vi "3HeClose.vi"(8 "error in (no error)":errorcluster, 11 "VISA resource name":refnum<visa-resource-name>) -> (0 "error out":errorcluster)   [LabVIEW 2018]
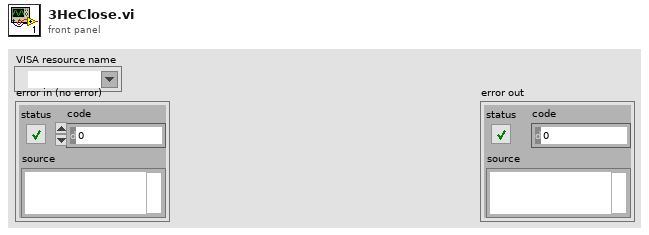
[diagram p1: front panel]
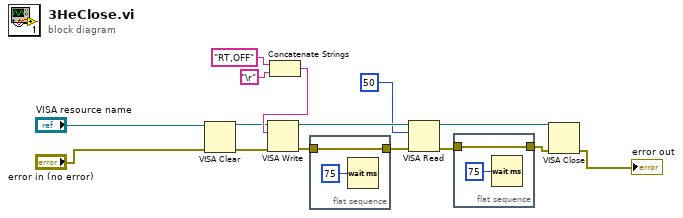
[diagram p0: block diagram]
diagram:
  n1 = VISA Clear(VISA resource name="VISA resource name", error in (no error)="error in (no error)") -> (VISA resource name out=w8:refnum<visa-resource-name>, error out=w9:errorcluster)
  n2 = Concatenate Strings("RT,OFF" ("write buffer"), "\r") -> (w10:string)
  n3 = VISA Write(VISA resource name=w8, write buffer=w10, error in (no error)=w9) -> (VISA resource name out=w14:refnum<visa-resource-name>, error out=w15:errorcluster)  [unwired: 1 out]
  n4 = flat-sequence {
    tunnel: w15 -> [w16]
    tunnel: [w16] -> w13
    frame #0 {
      n5 = Wait (ms)(milliseconds to wait=u32 75) -> ()  [unwired: 1 out]
    }
  }
  n6 = VISA Read(VISA resource name=w14, byte count=u32 50, error in (no error)=w13) -> (VISA resource name out=w3:refnum<visa-resource-name>, error out=w5:errorcluster)  [unwired: 2 out]
  n7 = flat-sequence {
    tunnel: w5 -> [w18]
    tunnel: [w18] -> w4
    frame #0 {
      n8 = Wait (ms)(milliseconds to wait=u32 75) -> ()  [unwired: 1 out]
    }
  }
  n9 = VISA Close(VISA resource name=w3, error in (no error)=w4) -> (error out=→"error out":errorcluster)
